vi "Read Multi-Point [MP].vi"(8 "error in (no error)":errorcluster, 9 "array size":i32, 10 "maximum time (5s)":dbl[unit]=5000.0 caption="maximum time (5000 ms)", 11 "CS++DMM in":refnum<class "CS++DMM.lvclass">) -> (0 "error out":errorcluster, 1 "actual number of points":i32, 2 "reading array":dbl[](array[numeric]) format="%^.2e", 3 "CS++DMM out":refnum<class "CS++DMM.lvclass">)   [LabVIEW 2013, in "CS++DMM.lvlib" / "CS++DMM.lvclass"]
doc: "This VI initiates the measurement, waits for the DMM to return to the Idle state, and returns an array of measured values. The number of measurements the DMM takes is determined by the values you specify for the Trigger Count and Sample Count parameters of the IviDmm Configure Multi-Point [MP] VI.\n\nThis VI applies default values to properties that have not been set by the user under the following conditions:\n\n(1) If the user has not set the value of any property in the IviDmmMultiPoint extension group, the VI sets the IviDmm>>Multi-Point Acquisition>>Sample Count [MP] and IviDmm>>Multi-Point Acquisition>>Trigger Count [MP] properties to 1.\n\n(2) If the user has not set the value of the IviDmm>Measurement Operation Options>Auto Zero [AZ] property, the VI sets the value of this property to IVIDMM_VAL_AUTO_ZERO_OFF (0). \n\nNotes:\n\n(1) This VI is part of the IviDmmMultiPoint [MP] extension group.\n\n(2) After this VI executes, each element in the Reading Array parameter is an actual reading or a value indicating that an over-range condition occurred.\n\n(3) If an over-range condition occurs, the corresponding Reading Array element contains an IEEE defined NaN (Not a Number) value and the VI returns the IVIDMM_WARN_OVER_RANGE (0x3FFA2001) warning code. \n\n(4) You can test each element in the Reading Array parameter for an over-range condition by calling the IviDmm Is Over-Range VI.\n\n(5) This VI performs interchangeability checking when the IviDmm>>Inherent IVI Settings>>User Options>>Interchange Check property is set to TRUE. If the IviDmm>>Inherent IVI Settings>>User Options>>Spy property is set to TRUE, you use the NI Spy utility to view interchangeability warnings. You use the IviDmm Get Next Interchange Warning VI to retrieve interchangeability warnings when the IviDmm>>Inherent IVI Settings>>User Options>>Spy property is set to FALSE. For more information about interchangeability checking, refer to the help text for the IviDmm>>Inherent IVI Settings>>User Options>>Interchange Check property.\n\n(6) The class driver initiates an array of simulated measurements when this VI is called and the IviDmm>>Inherent IVI Settings>>User Options>>Simulate property is set to TRUE and the IviDmm>>Inherent IVI Settings>>User Options>>Use Specific Simulation property is set to FALSE. For information on how to configure a simulated measurement, refer to the online help manual."
uses:
  CS++DMM.lvclass
  CS++DMM.lvclass/CS++DMM.ctl
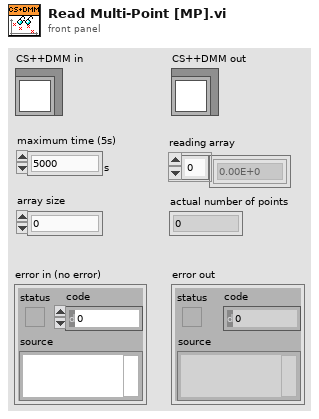
[diagram p1: front panel]
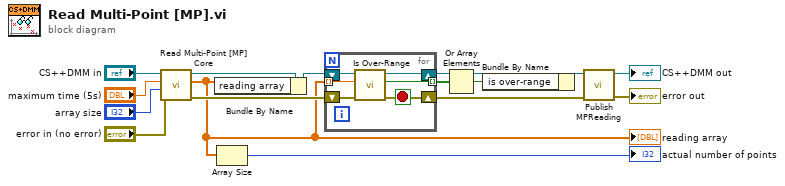
[diagram p0: block diagram]
diagram:
  n1 = call-dynamic "Read Multi-Point [MP] Core.vi"("error in (no error)"="error in (no error)", "array size"="array size", "maximum time (5s)"="maximum time (5s)", "CS++DMM in"="CS++DMM in") -> ("error out"=w7:errorcluster, "reading array"=w3:dbl[], "CS++DMM out"=w10:refnum<class "CS++DMM.lvclass">)  [unwired: 4 in, 1 out]
  "reading array" <- w3
  n2 = Bundle By Name(cluster=w10, "reading array"=w3) -> (w6:refnum<class "CS++DMM.lvclass">)
  n3 = Array Size(array=w3) -> (size(s)=→"actual number of points":i32)
  n4 = for {
    tunnel: [w22] -> w8 mode=indexing
    tunnel: w3 -> [w18] mode=indexing
    shift-right: [w19] -> w5
    shift-left: w6 -> [w20]
    shift-right: [w17] -> w1
    shift-left: w7 -> [w21]
    stop <- w17 stop-if-true
    n5 = call-dynamic "Is Over-Range.vi"("error in (no error)"=w21, "measurement value"=w18, "CS++DMM in"=w20) -> ("error out"=w17:errorcluster, "is over-range"=w22:bool, "CS++DMM out"=w19:refnum<class "CS++DMM.lvclass">)  [unwired: 6 in]
  }
  n6 = Or Array Elements(Boolean array=w8) -> (logical OR=w2:bool)
  n7 = Bundle By Name(cluster=w5, "is over-range"=w2) -> (w4:refnum<class "CS++DMM.lvclass">)
  n8 = call "Publish MPReading.vi"("error in (no error)"=w1, "CS++DMM in"=w4) -> ("error out"=→"error out":errorcluster, "CS++DMM out"=→"CS++DMM out":refnum<class "CS++DMM.lvclass">)  [unwired: 8 in]
